vi "Move.vi"(8 "error in (no error)":errorcluster, 10 "Amount (rev)":dbl, 11 "Dummy Motor in":refnum<class "Dummy Motor.lvclass">) -> (0 "error out":errorcluster, 3 "Dummy Motor out":refnum<class "Dummy Motor.lvclass">)   [LabVIEW 2019, in "Dummy Motor.lvclass"]
uses:
  Dummy Motor.lvclass
  Dummy Motor.lvclass/Dummy Motor.ctl
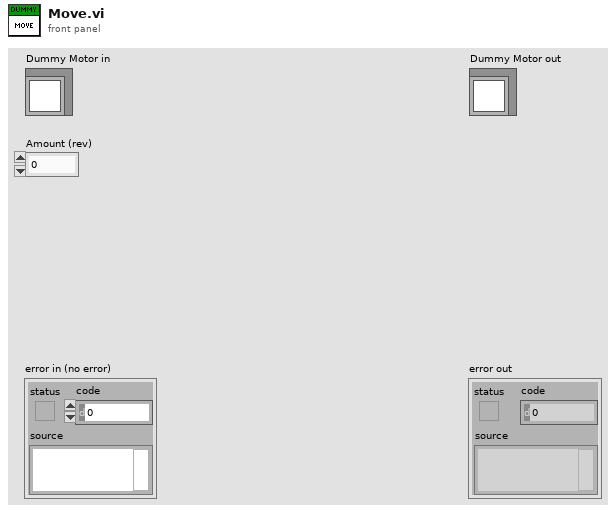
[diagram p1: front panel]
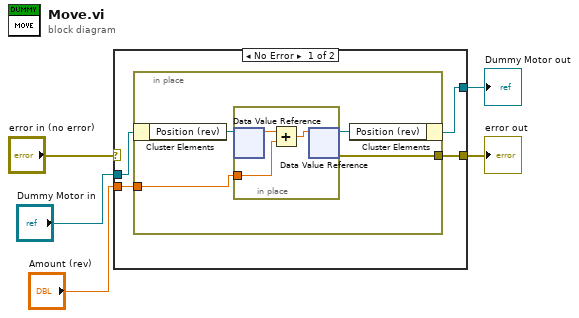
[diagram p0: block diagram]
diagram:
  n1 = case shown="No Error" "error in (no error)" {
    selector: "error in (no error)" -> [_ w18]
    tunnel: [w6 w18] -> w3
    tunnel: [w8 w17] -> w2
    tunnel: "Dummy Motor in" -> [w9 w17]
    tunnel: "Amount (rev)" -> [w7 _]
    frame No Error {
      n2 = in-place {
        in-place-border: w7 -> [w10]
        in-place-border: [w11] -> w6
        n3 = in-place-cluster #1(w9) -> ("Position (rev)"=w13:refnum<data-value>)
        n4 = in-place {
          in-place-border: w10 -> [w15]
          n5 = in-place-dvr #2(w13) -> (w16:dbl)  [unwired: 1 out]
          n6 = Add(x=w16, y=w15) -> (x+y=w14:dbl)
          n7 = in-place-dvr #2(w14) -> (w12:refnum<data-value>, w11:errorcluster)
        }
        n8 = in-place-cluster #1("Position (rev)"=w12) -> (w8:refnum<class "Dummy Motor.lvclass">)
      }
    }
    frame Error {
    }
  }
  "error out" <- w3
  "Dummy Motor out" <- w2
